vi "Read Interface.vi"(8 "error in (no error)":errorcluster, 11 "CAN_RW_CORE in":refnum<class "L2ENET_RW_CORE.lvclass">) -> (0 "error out":errorcluster, 2 "Interface":string, 3 "CAN_RW_CORE out":refnum<class "L2ENET_RW_CORE.lvclass">)   [LabVIEW 2021, in "L2ENET_RW_CORE.lvclass"]
uses:
  L2ENET_RW_CORE.lvclass
  L2ENET_RW_CORE.lvclass/L2ENET_RW_CORE.ctl
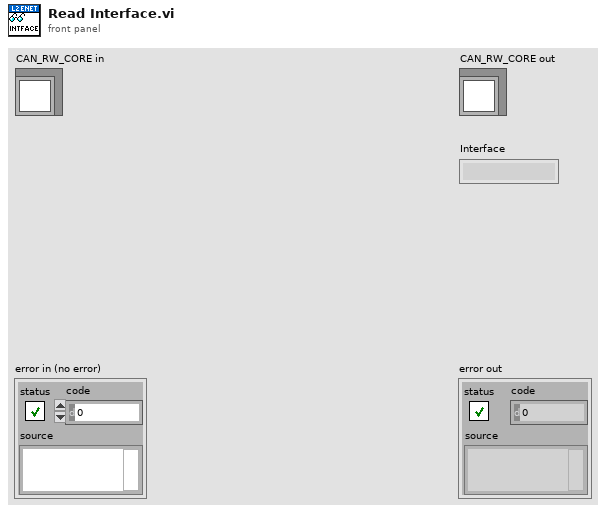
[diagram p1: front panel]
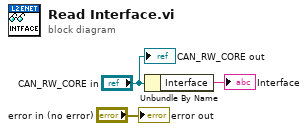
[diagram p0: block diagram]
diagram:
  n1 = Unbundle By Name("CAN_RW_CORE in") -> ("Interface"=→"Interface":string)
  "error out" <- "error in (no error)"
  "CAN_RW_CORE out" <- "CAN_RW_CORE in"
